vi "Filter.vi"(8 "error in (no error)":errorcluster, 11 "Software Lock-in in":refnum<class "Software Lock-in.lvclass">) -> (0 "error out":errorcluster, 3 "Software Lock-in out":refnum<class "Software Lock-in.lvclass">)   [LabVIEW 2016, in "Software Lock-in.lvclass"]
uses:
  Software Lock-in.lvclass
  Software Lock-in.lvclass/Software Lock-in.ctl
  Utilities/Fit/Smooth Background CDBL.vi
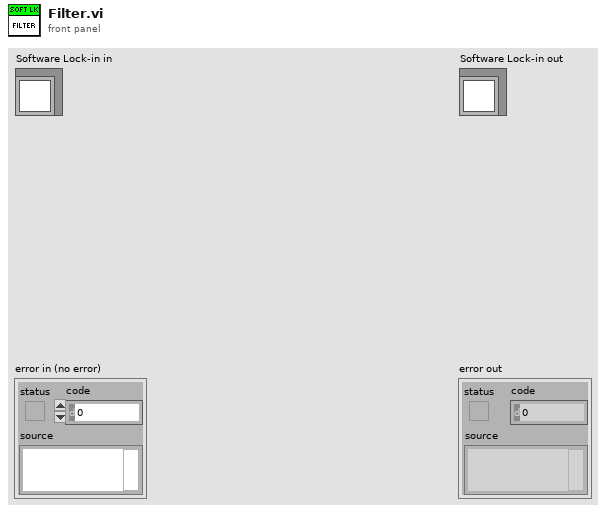
[diagram p1: front panel]
types:
  T1 = enum16{"Lowpass", "Highpass", "Bandpass", "Bandstop"}
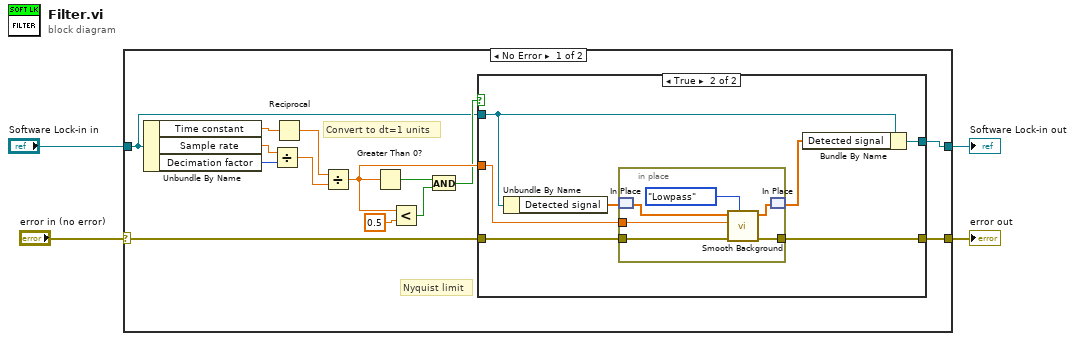
[diagram p0: block diagram]
diagram:
  n1 = case shown="No Error" "error in (no error)" {
    selector: "error in (no error)" -> [w7 w35]
    tunnel: [w6 w35] -> w3
    tunnel: [w8 w34] -> w1
    tunnel: "Software Lock-in in" -> [w9 w34]
    frame No Error {
      # "Convert to dt=1 units"
      # "Nyquist limit"
      n2 = Unbundle By Name(w9) -> ("Time constant"=w5:dbl, "Sample rate"=w18:dbl, "Decimation factor"=w17:i32)
      n3 = Divide(x=w18, y=w17) -> (x/y=w15:dbl)
      n4 = Reciprocal(x=w5) -> (1/x=w16:dbl)
      n5 = Divide(x=w16, y=w15) -> (x/y=w12:dbl)
      n6 = Greater Than 0?(x=w12) -> (x > 0?=w10:bool)
      n7 = Less?(x=w12, y=0.5) -> (x < y?=w13:bool)
      n8 = And(x=w10, y=w13) -> (x .and. y?=w11:bool)
      n9 = case shown="True" w11 {
        tunnel: w12 -> [_ w27]
        tunnel: w7 -> [w19 w26]
        tunnel: w9 -> [w20 w24]
        tunnel: [w20 w23] -> w8
        tunnel: [w19 w21] -> w6
        frame False {
        }
        frame True {
          n10 = Unbundle By Name(w24) -> ("Detected signal"=w25:cdb[])
          n11 = in-place {
            in-place-border: w26 -> [w30]
            in-place-border: [w31] -> w21
            in-place-border: w27 -> [w28]
            n12 = in-place-match #1(w25) -> (w33:cdb[])
            n13 = call-poly "Smooth Background.vi"("Type"=T1."Lowpass", "Error In"=w30, "LP  F"=w28, "Data"=w33) -> ("Error Out"=w31:errorcluster, "Data out"=w32:cdb[])  [unwired: 6 in]
            n14 = in-place-match #1(w32) -> (w22:cdb[])
          }
          n15 = Bundle By Name(cluster=w24, "Detected signal"=w22) -> (w23:refnum<class "Software Lock-in.lvclass">)
        }
      }
    }
    frame Error {
    }
  }
  "error out" <- w3
  "Software Lock-in out" <- w1
